vi "Stop_Watch.vi"(0 "SW_Controller":T1) -> (4 "ms":T2[](array[typedef]))   [LabVIEW 2021]
doc: "This VI is a digital stop watch, which does the Same operations of normal Stop watches."
uses:
  Controls/SR_Constants.ctl
  Controls/7_Segment_Display.ctl
  Controls/SW_Controller.ctl
panel:
  out "Colon6":bool
  out "Colon1":bool
  out "Colon5":bool
  out "Colon2":bool
  out "Colon4":bool
  out "Colon3":bool
  out "Sec":T2[](array[typedef])
  out "Min":T2[](array[typedef])
  out "Hour":T2[](array[typedef])
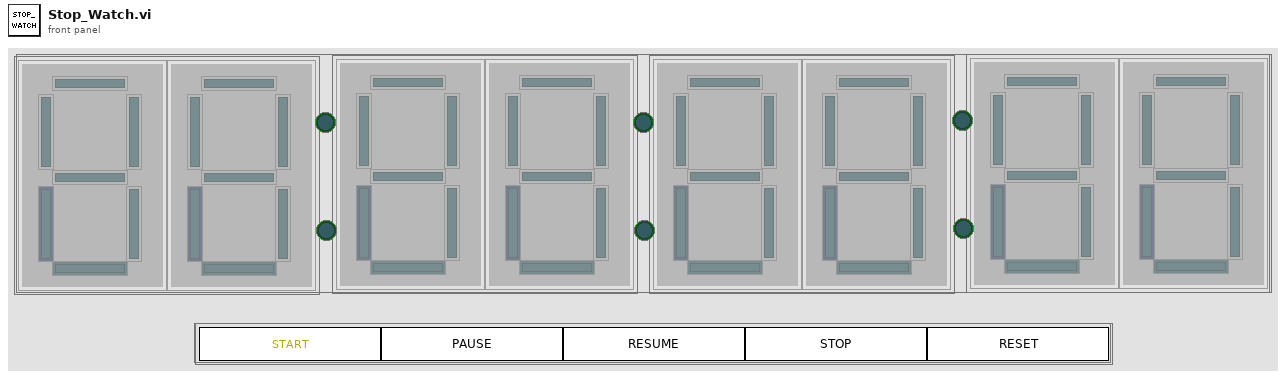
[diagram p1: front panel]
types:
  T1 = typedef "SW_Controller.ctl" = cluster{"Start":bool, "Pause":bool, "Resume":bool, "Stop":bool, "Reset":bool}
  T2 = typedef "7_Segment_Display.ctl" = cluster{"a":bool, "b":bool, "c":bool, "d":bool, "e":bool, "f":bool, "g":bool}
  T3 = typedef "SR_Constants.ctl" = cluster{"Stop_Watch_Time":dbl, "SW_Start_Time":dbl, "Pause?":bool, "Stop?":bool}
  T4 = typedef "Time_Format.ctl" = cluster{"Hours":i32, "Min":i32, "Sec":i32, "ms":i32}
  T5 = enum16{"Left Button", "Center Button", "Right Button", "Window Close"}
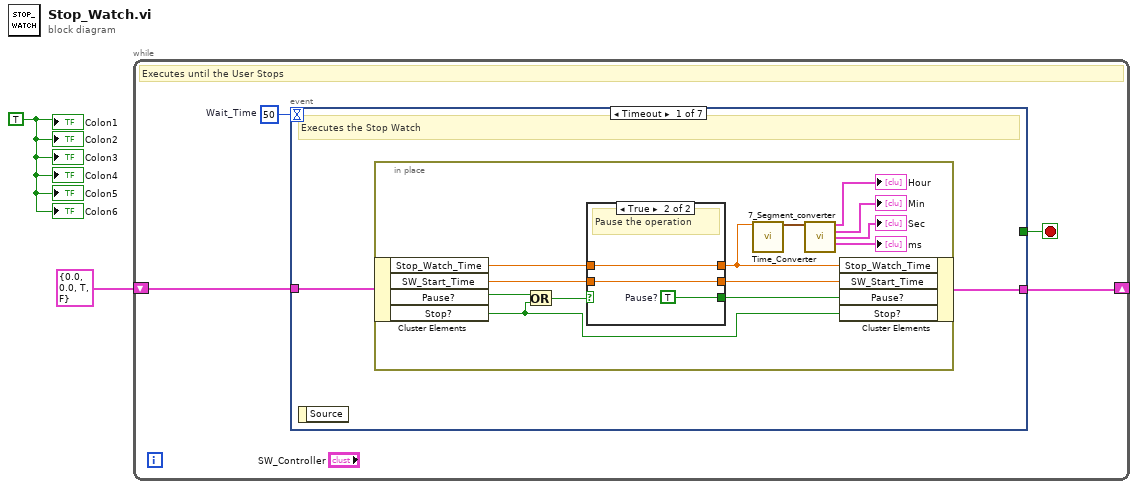
[diagram p0: block diagram]
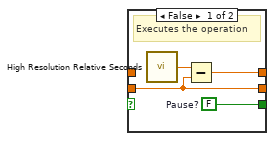
[diagram p2: hidden frame]
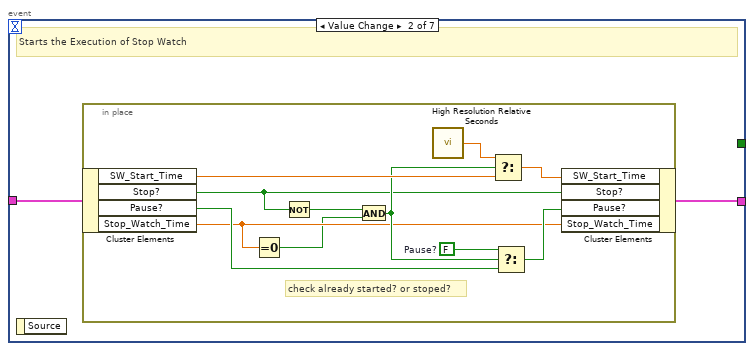
[diagram p3: hidden frame]
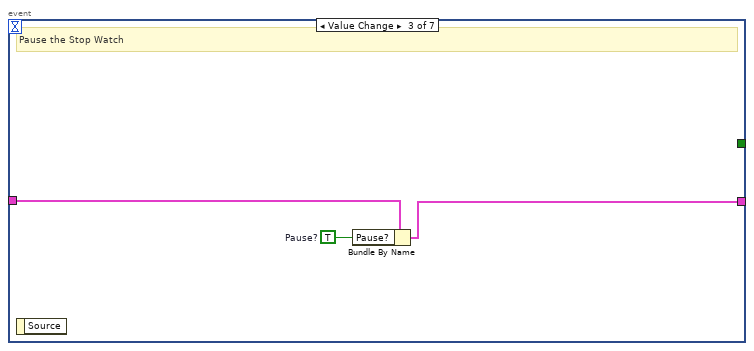
[diagram p4: hidden frame]
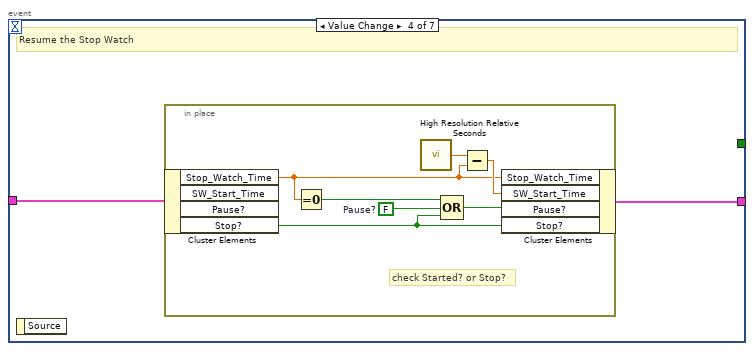
[diagram p5: hidden frame]
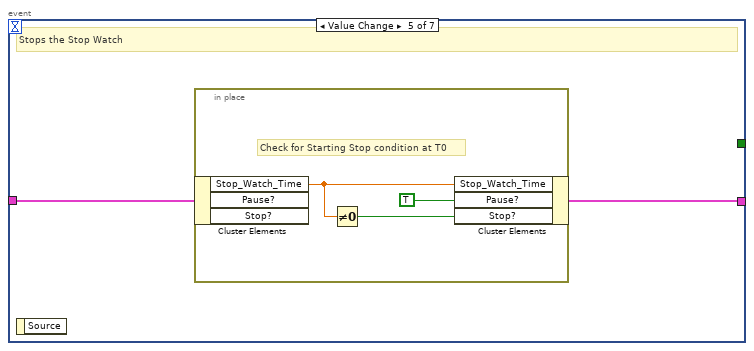
[diagram p6: hidden frame]
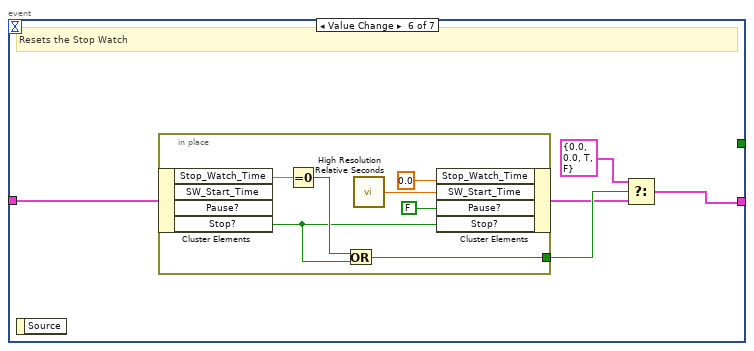
[diagram p7: hidden frame]
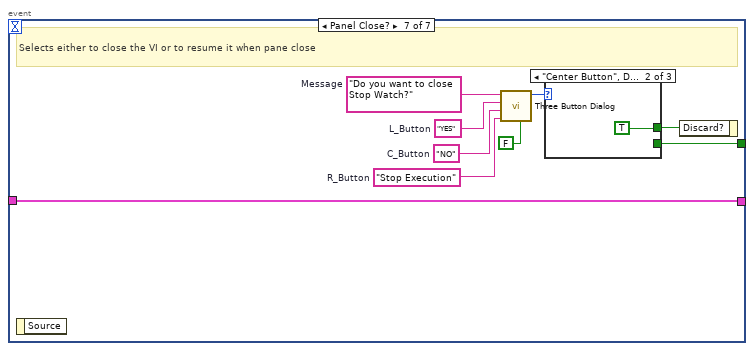
[diagram p8: hidden frame]
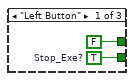
[diagram p9: hidden frame]
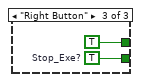
[diagram p10: hidden frame]
diagram:
  w1 = TRUE
  n1 = while {
    shift-right: [w4] -> _
    shift-left: T3 {"Stop_Watch_Time"=0.0, "SW_Start_Time"=0.0, "Pause?"=TRUE, "Stop?"=FALSE} -> [w5]
    stop <- w3 stop-if-true
    w6 = 50  # Wait_Time
    # "Executes until the User Stops"
    n2 = event "Selescts the operations" shown="[0] Timeout" {
      selector: _ -> [_ _ _ _ _ _ _]
      dyn-events: _ -> [_ _ _ _ _ _ _]
      timeout: w6 -> [_ _ _ _ _ _ _]
      tunnel: w5 -> [w8 w29 w44 w46 w55 w63 w79]
      tunnel: [w7 w30 w43 w45 w54 w59 w79] -> w4
      tunnel: [_ _ _ _ _ _ w71] -> w3
      event Timeout {
        # "Executes the Stop Watch"
        n3 = event-data() -> ()  [unwired: 1 in, 1 out]
        n4 = in-place "In Place Element Structure" {
          n5 = in-place-cluster #1(w8) -> ("Stop_Watch_Time"=w21:dbl, "SW_Start_Time"=w20:dbl, "Pause?"=w16:bool, "Stop?"=w14:bool)
          n6 = Or(x=w16, y=w14) -> (x .or. y?=w15:bool)
          n7 = case shown="True" w15 {
            tunnel: [w25 w28] -> w17
            tunnel: w20 -> [w24 w27]
            tunnel: [w24 w27] -> w18
            tunnel: [w23 w26] -> w19
            tunnel: w21 -> [_ w26]
            frame False {
              w25 = FALSE  # Pause?
              # "Executes the operation"
              n8 = call <vilib>:"High Resolution Relative Seconds.vi"() -> ("relative seconds"=w22:dbl)
              n9 = Subtract(x=w22, y=w24) -> (x-y=w23:dbl)
            }
            frame True {
              w28 = TRUE  # Pause?
              # "Pause the operation"
            }
          }
          n10 = call "Time_Converter.vi"("Stop_Watch_Time"=w19) -> ("Time_Format"=w13:T4)  [unwired: 14 in]
          n11 = call "7_Segment_converter.vi"("Time_Format"=w13) -> ("Hours"=→"Hour":T2[], "Min"=→"Min":T2[], "Sec"=→"Sec":T2[], "ms"=→"ms":T2[])  [unwired: 11 in]
          n12 = in-place-cluster #1("Stop_Watch_Time"=w19, "SW_Start_Time"=w18, "Pause?"=w17, "Stop?"=w14) -> (w7:T3)
        }
      }
      event Value Change {
        # "Starts the Execution of Stop Watch"
        n13 = event-data() -> ()  [unwired: 1 in, 1 out]
        n14 = in-place "In Place Element Structure" {
          w40 = FALSE  # Pause?
          # "check already started? or stoped?"
          n15 = in-place-cluster #2(w29) -> ("SW_Start_Time"=w39:dbl, "Stop?"=w31:bool, "Pause?"=w35:bool, "Stop_Watch_Time"=w34:dbl)
          n16 = Equal To 0?(x=w34) -> (x = 0?=w32:bool)
          n17 = Not(x=w31) -> (.not. x?=w33:bool)
          n18 = And(x=w33, y=w32) -> (x .and. y?=w37:bool)
          n19 = call <vilib>:"High Resolution Relative Seconds.vi"() -> ("relative seconds"=w41:dbl)
          n20 = Select(t=w41, s=w37, f=w39) -> (s? t:f=w38:dbl)
          n21 = Select(t=w40, s=w37, f=w35) -> (s? t:f=w36:bool)
          n22 = in-place-cluster #2("SW_Start_Time"=w38, "Stop?"=w31, "Pause?"=w36, "Stop_Watch_Time"=w34) -> (w30:T3)
        }
      }
      event Value Change {
        w42 = TRUE  # Pause?
        # "Pause the Stop Watch"
        n23 = event-data() -> ()  [unwired: 1 in, 1 out]
        n24 = Bundle By Name(cluster=w44, "Pause?"=w42) -> (w43:T3)
      }
      event Value Change {
        # "Resume the Stop Watch"
        n25 = event-data() -> ()  [unwired: 1 in, 1 out]
        n26 = in-place "In Place Element Structure" {
          w52 = FALSE  # Pause?
          # "check Started? or Stop?"
          n27 = in-place-cluster #3(w46) -> ("Stop_Watch_Time"=w49:dbl, "Stop?"=w47:bool)  [unwired: 2 out]
          n28 = Equal To 0?(x=w49) -> (x = 0?=w51:bool)
          n29 = call <vilib>:"High Resolution Relative Seconds.vi"() -> ("relative seconds"=w53:dbl)
          n30 = Compound Arithmetic op=OR(w51, w52, w47) -> (w48:bool)
          n31 = Subtract(x=w53, y=w49) -> (x-y=w50:dbl)
          n32 = in-place-cluster #3("Stop_Watch_Time"=w49, "SW_Start_Time"=w50, "Pause?"=w48, "Stop?"=w47) -> (w45:T3)
        }
      }
      event Value Change {
        # "Stops the Stop Watch"
        n33 = event-data() -> ()  [unwired: 1 in, 1 out]
        n34 = in-place "In Place Element Structure" {
          # "Check for Starting Stop condition at T0"
          n35 = in-place-cluster #4(w55) -> ("Stop_Watch_Time"=w58:dbl)  [unwired: 2 out]
          n36 = Not Equal To 0?(x=w58) -> (x != 0?=w56:bool)
          n37 = in-place-cluster #4("Stop_Watch_Time"=w58, "Pause?"=TRUE, "Stop?"=w56) -> (w54:T3)
        }
      }
      event Value Change {
        # "Resets the Stop Watch"
        n38 = event-data() -> ()  [unwired: 1 in, 1 out]
        n39 = in-place "In Place Element Structure" {
          in-place-border: [w64] -> w62
          n40 = in-place-cluster #5(w63) -> ("Stop_Watch_Time"=w67:dbl, "Stop?"=w65:bool)  [unwired: 2 out]
          n41 = Equal To 0?(x=w67) -> (x = 0?=w66:bool)
          n42 = Or(x=w66, y=w65) -> (x .or. y?=w64:bool)
          n43 = call <vilib>:"High Resolution Relative Seconds.vi"() -> ("relative seconds"=w69:dbl)
          n44 = in-place-cluster #5("Stop_Watch_Time"=0.0, "SW_Start_Time"=w69, "Pause?"=FALSE, "Stop?"=w65) -> (w60:T3)
        }
        n45 = Select(t=T3 {"Stop_Watch_Time"=0.0, "SW_Start_Time"=0.0, "Pause?"=TRUE, "Stop?"=FALSE}, s=w62, f=w60) -> (s? t:f=w59:T3)
      }
      event Panel Close? {
        w76 = "Stop Execution"  # R_Button
        w75 = "NO"  # C_Button
        w77 = "YES"  # L_Button
        w78 = "Do you want to close Stop Watch?"  # Message
        # "Selects either to close the VI or to resume it when pane close"
        n46 = event-data() -> ()  [unwired: 1 in, 1 out]
        n47 = call <vilib>:"Three Button Dialog.vi"("Allow user to close window? (TRUE)"=FALSE, "Right Button Text (\"Cancel\")"=w76, "Center Button Text (\"No\")"=w75, "Left Button Text (\"Yes\")"=w77, "message"=w78) -> ("Which Button?"=w73:T5)  [unwired: 6 in]
        n48 = case shown="\"Center Button\", Default" w73 {
          tunnel: [FALSE TRUE TRUE] -> w72
          tunnel: [w80 _ w83] -> w71
          frame "Left Button" {
            w80 = TRUE  # Stop_Exe?
          }
          frame "Center Button", Default {
          }
          frame "Right Button" {
            w83 = TRUE  # Stop_Exe?
          }
        }
        n49 = event-data ("Event Filter Node")("Discard?"=w72) -> ()  [unwired: 1 in, 1 out]
      }
    }
  }
  "Colon3" <- w1
  "Colon4" <- w1
  "Colon2" <- w1
  "Colon1" <- w1
  "Colon5" <- w1
  "Colon6" <- w1
